vi "CheckMove.vi"(1 "col":i32, 2 "Board":i32[][](array[numeric])) -> (0 "Valid":bool)   [LabVIEW 2025]
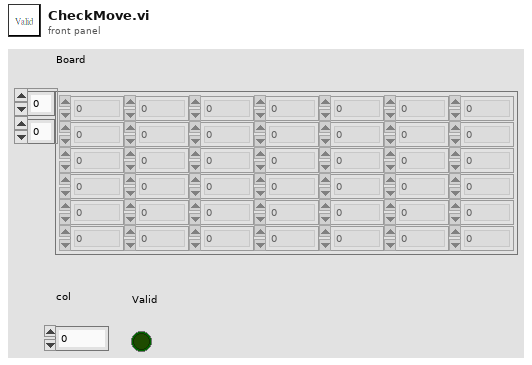
[diagram p1: front panel]
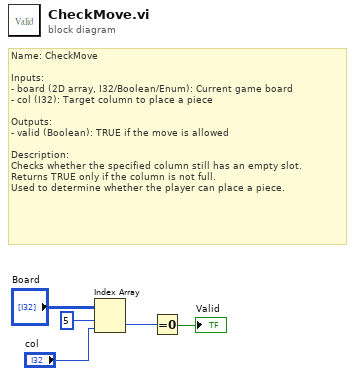
[diagram p0: block diagram]
diagram:
  # "Name: CheckMove\n\nInputs:\n- board (2D array, I32/Boolean/Enum): Current game board\n- col (I32): Target column to place a piece\n\nOutputs:\n- valid (Boolean): TRUE if the move is allowed\n\nDescription:\nChecks whether the specified column still has an empty slot.\nReturns TRUE only if the column is not full.\nUsed to determine whether the player can place a piece."
  n1 = Index Array(array="Board", index (row)=5, index (col)="col") -> (element=w5:i32)
  n2 = Equal To 0?(x=w5) -> (x = 0?=→"Valid":bool)
